vi "Loop Get Input Output Assignements.vi"(10 "Inside Terms[] offset":i32, 11 "Loop Tunnels[]":refnum<vi>[](array[refnum])) -> (2 "Output assignements":string, 3 "Input assignements":string)   [LabVIEW 2014]
doc: "Return C code assignement for getting input values from outside into Loop and also assign values to outside wires.\nInside Terms[] offset is for multiframe structures (CaseStructure),it's used when parsing tunnels to use right internal terminal, because each outside terminal has N inside terminals (N is count of structure frames)."
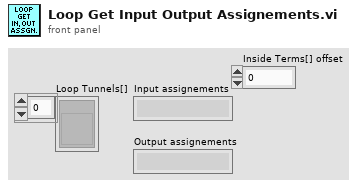
[diagram p1: front panel]
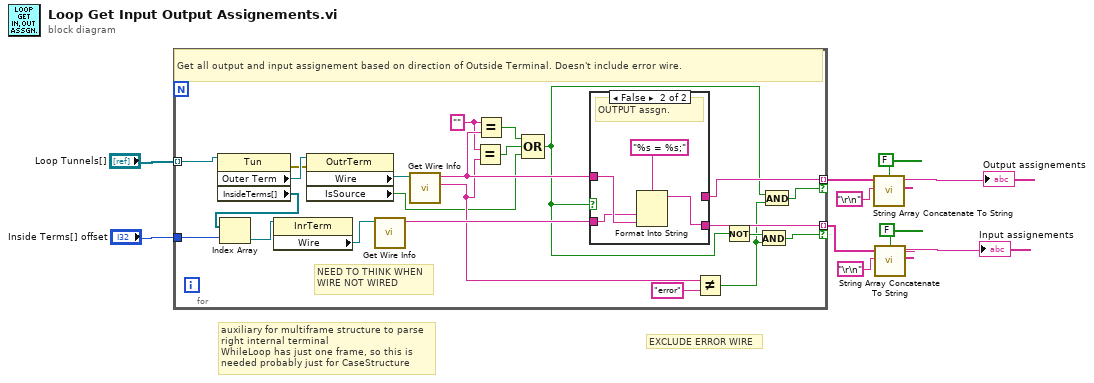
[diagram p0: block diagram]
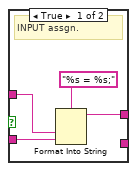
[diagram p2: hidden frame]
diagram:
  # "auxiliary for multiframe structure to parse right internal terminal\nWhileLoop has just one frame, so this is needed probably just for CaseStructure"
  # "EXCLUDE ERROR WIRE"
  n1 = for {
    tunnel: "Loop Tunnels[]" -> [w31] mode=indexing
    tunnel: [w25] -> w8 mode=indexing if=w23
    tunnel: [w24] -> w7 mode=indexing if=w22
    tunnel: "Inside Terms[] offset" -> [w18]
    w15 = "" ("x")
    # "NEED TO THINK WHEN WIRE NOT WIRED"
    # "Get all output and input assignement based on direction of Outside Terminal. Doesn't include error wire."
    n2 = property class="Tun"(reference=w31) -> (error out=w32:errorcluster, "Outer Term"=w33:refnum<vi>, "InsideTerms[]"=w29:refnum<vi>[])  [unwired: 1 in, 1 out]
    n3 = Index Array(array=w29, index=w18) -> (element=w28:refnum<vi>)
    n4 = property class="InrTerm"(reference=w28) -> ("Wire"=w27:refnum<vi>)  [unwired: 1 in, 2 out]
    n5 = property class="OutrTerm"(reference=w33, error in=w32) -> ("Wire"=w30:refnum<vi>, "IsSource"=w12:bool)  [unwired: 2 out]
    n6 = call "Get Wire Info.vi"("Wire"=w27) -> ("wire label"=w26:string)  [unwired: 9 in, 1 out]
    n7 = call "Get Wire Info.vi"("Wire"=w30) -> ("wire datatype"=w16:string, "wire label"=w17:string)  [unwired: 9 in]
    n8 = Equal?(x=w15, y=w16) -> (x = y?=w13:bool)
    n9 = Equal?(x=w15, y=w17) -> (x = y?=w14:bool)
    n10 = Compound Arithmetic op=OR(w14, w13, w12) -> (w11:bool)
    n11 = case shown="False" w11 {
      tunnel: w17 -> [w36 w40]
      tunnel: w26 -> [w35 w39]
      tunnel: [w34 _] -> w25
      tunnel: [_ w38] -> w24
      frame True {
        # "INPUT assgn."
        n12 = Format Into String(format string="%s = %s;", w36, w35) -> (resulting string=w34:string)  [unwired: 2 in, 1 out]
      }
      frame False {
        # "OUTPUT assgn."
        n13 = Format Into String(format string="%s = %s;", w39, w40) -> (resulting string=w38:string)  [unwired: 2 in, 1 out]
      }
    }
    n14 = Not Equal?(x=w16, y="error") -> (x != y?=w20:bool)
    n15 = Not(x=w11) -> (.not. x?=w21:bool)
    n16 = And(x=w21, y=w20) -> (x .and. y?=w22:bool)
    n17 = And(x=w11, y=w20) -> (x .and. y?=w23:bool)
  }
  n18 = call "String Array Concatenate To String.vi"("insert last delimiter?"=FALSE, "Delimiter char"="\r\n", "Array String In"=w8) -> ("String"=→"Output assignements":string)  [unwired: 8 in]
  n19 = call "String Array Concatenate To String.vi"("insert last delimiter?"=FALSE, "Delimiter char"="\r\n", "Array String In"=w7) -> ("String"=→"Input assignements":string)  [unwired: 8 in]
